vi "empty_FIFO.vi"(8 "error in":errorcluster, 11 "Refnum in":T1) -> (0 "error out":errorcluster, 2 "Elements Remaining 2":u32, 3 "Refnum out":T1)   [LabVIEW 2017]
uses:
  controls/SS_fpga_sysID_REFTYPE.ctl
  <vilib>/Utility/error.llb/Error Cluster From Error Code.vi
  <vilib>/rvi/errors/niLvFpgaAdjustHostInterfaceError.vi
  <vilib>/rvi/interface/nirviMethod/nirviMethod.xnode
  FPGA Bitfiles/SS_fpga_swept_sines.lvbitx
  <vilib>/FPGAPlugInAG/cRIO-9082/niLvFpga_ReadFifo_cRIO-9082.vi
  <vilib>/rvi/errors/niLvFpgaMergeErrorWithErrorCode.vi
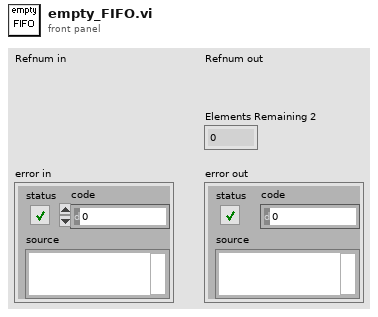
[diagram p1: front panel]
types:
  T1 = typedef "SS_fpga_sysID_REFTYPE.ctl" = refnum<k20>
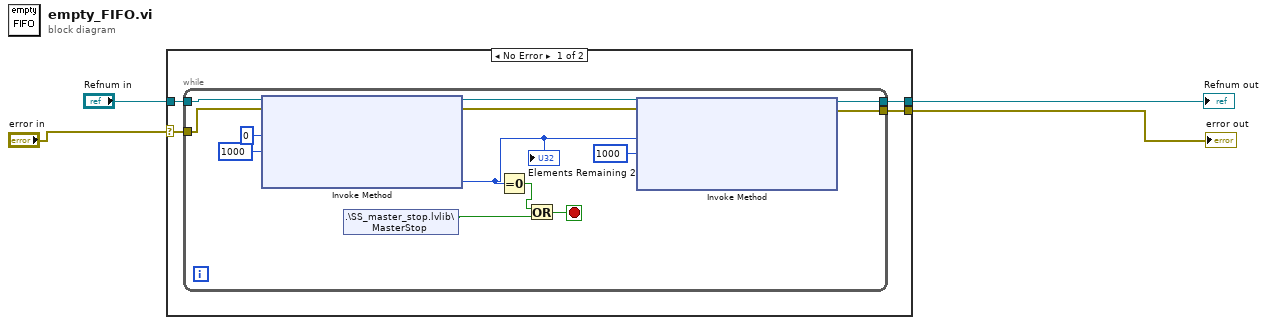
[diagram p0: block diagram]
diagram:
  n1 = case shown="No Error" "error in" {
    selector: "error in" -> [w5 w23]
    tunnel: [w8 w22] -> w4
    tunnel: [w7 w23] -> w3
    tunnel: "Refnum in" -> [w6 w22]
    frame No Error {
      n2 = while {
        tunnel: w6 -> [w21]
        tunnel: w5 -> [w14]
        tunnel: [w13] -> w8
        tunnel: [w12] -> w7
        stop <- w10 stop-if-true
        n3 = xnode "Invoke Method"("FPGA VI Reference In"=w21, "error in"=w14, "Number of Elements"=u32 0, "Timeout (ms)"=1000) -> ("FPGA VI Reference Out"=w19:T1, "error out"=w18:errorcluster, "Elements Remaining"=w17:u32)  [unwired: 1 out]
        "Elements Remaining 2" <- w17
        n4 = shared-variable ".\\SS_master_stop.lvlib\\MasterStop"() -> (w9:bool)  [unwired: 1 in, 1 out]
        n5 = Equal To 0?(x=w17) -> (x = 0?=w11:bool)
        n6 = Or(x=w11, y=w9) -> (x .or. y?=w10:bool)
        n7 = xnode "Invoke Method"("FPGA VI Reference In"=w19, "error in"=w18, "Number of Elements"=w17, "Timeout (ms)"=1000) -> ("FPGA VI Reference Out"=w13:T1, "error out"=w12:errorcluster)  [unwired: 2 out]
      }
    }
    frame Error {
    }
  }
  "Refnum out" <- w4
  "error out" <- w3
